vi "Cycling_No_DAQ_Tasks_RT - .5C - Test.vi"() -> ()   [LabVIEW 2020]
panel:
  out "PS Visa Out 3":refnum<visa-resource-name>
  out "PS error out 3":errorcluster
  in  "PS error in 3":errorcluster caption="PS error in (no error)"
  out "PS Visa Out 2":refnum<visa-resource-name>
  out "PS error out 2":errorcluster
  in  "PS error in 2":errorcluster caption="PS error in (no error)"
  out "PS error out":errorcluster
  out "PS Visa Out":refnum<visa-resource-name>
  in  "PS error in":errorcluster caption="PS error in (no error)"
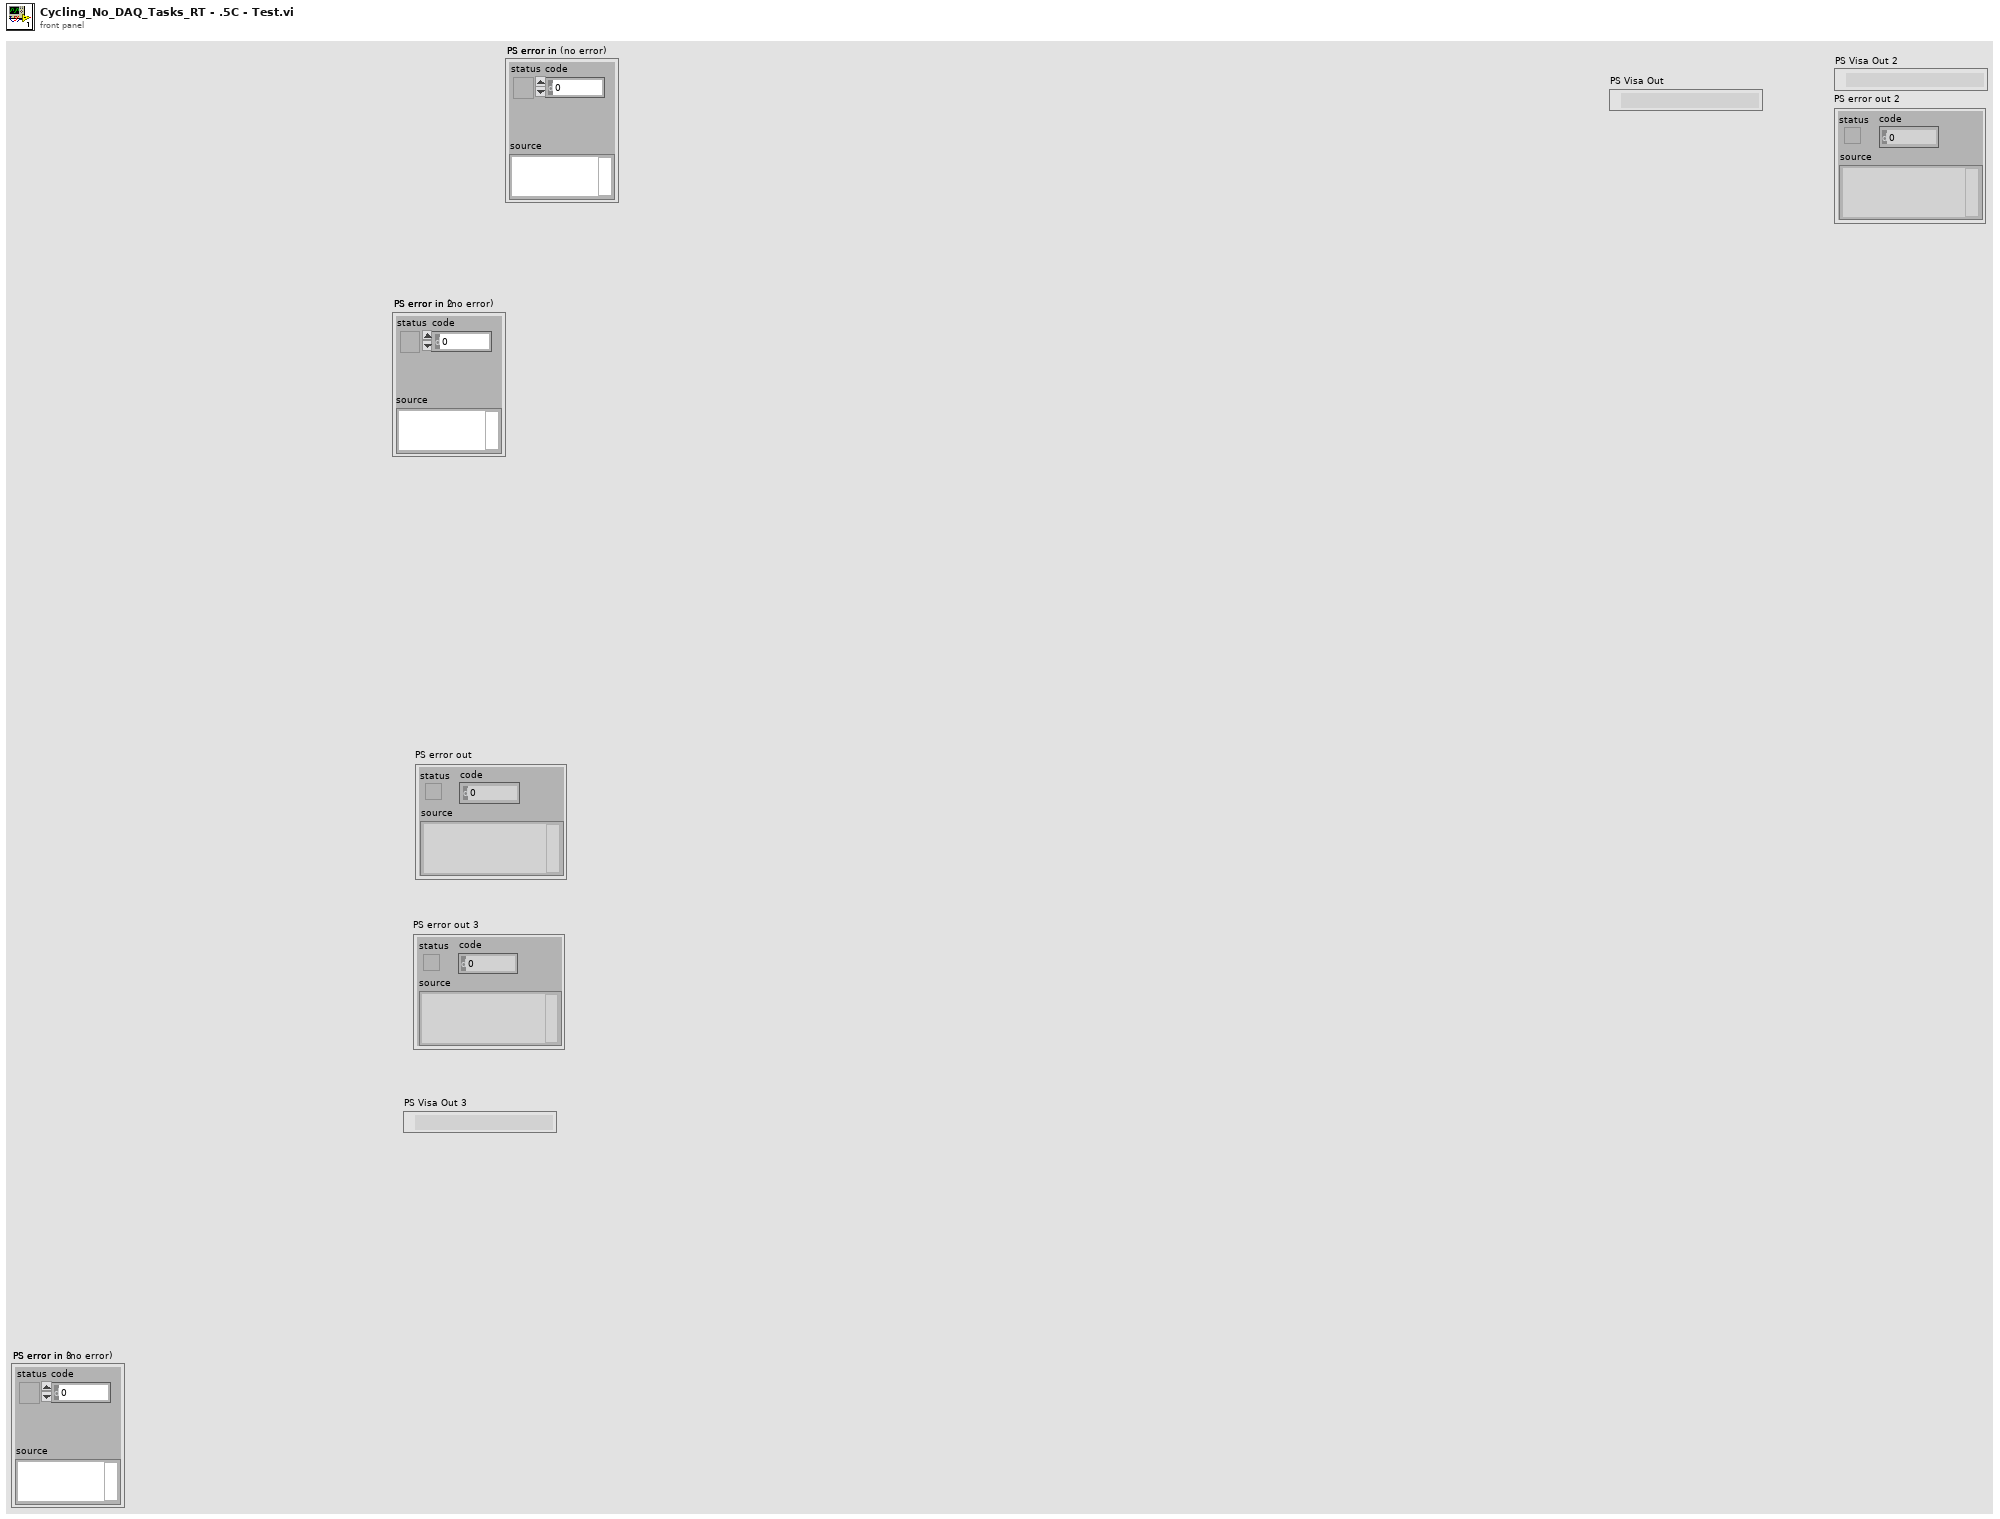
[diagram p1: front panel]
types:
  T1 = enum16{"\"30Q\"", "\"40T\"", "\"2P30Q\"", "\"3P30Q\"", "\"Nissan Leaf\""}
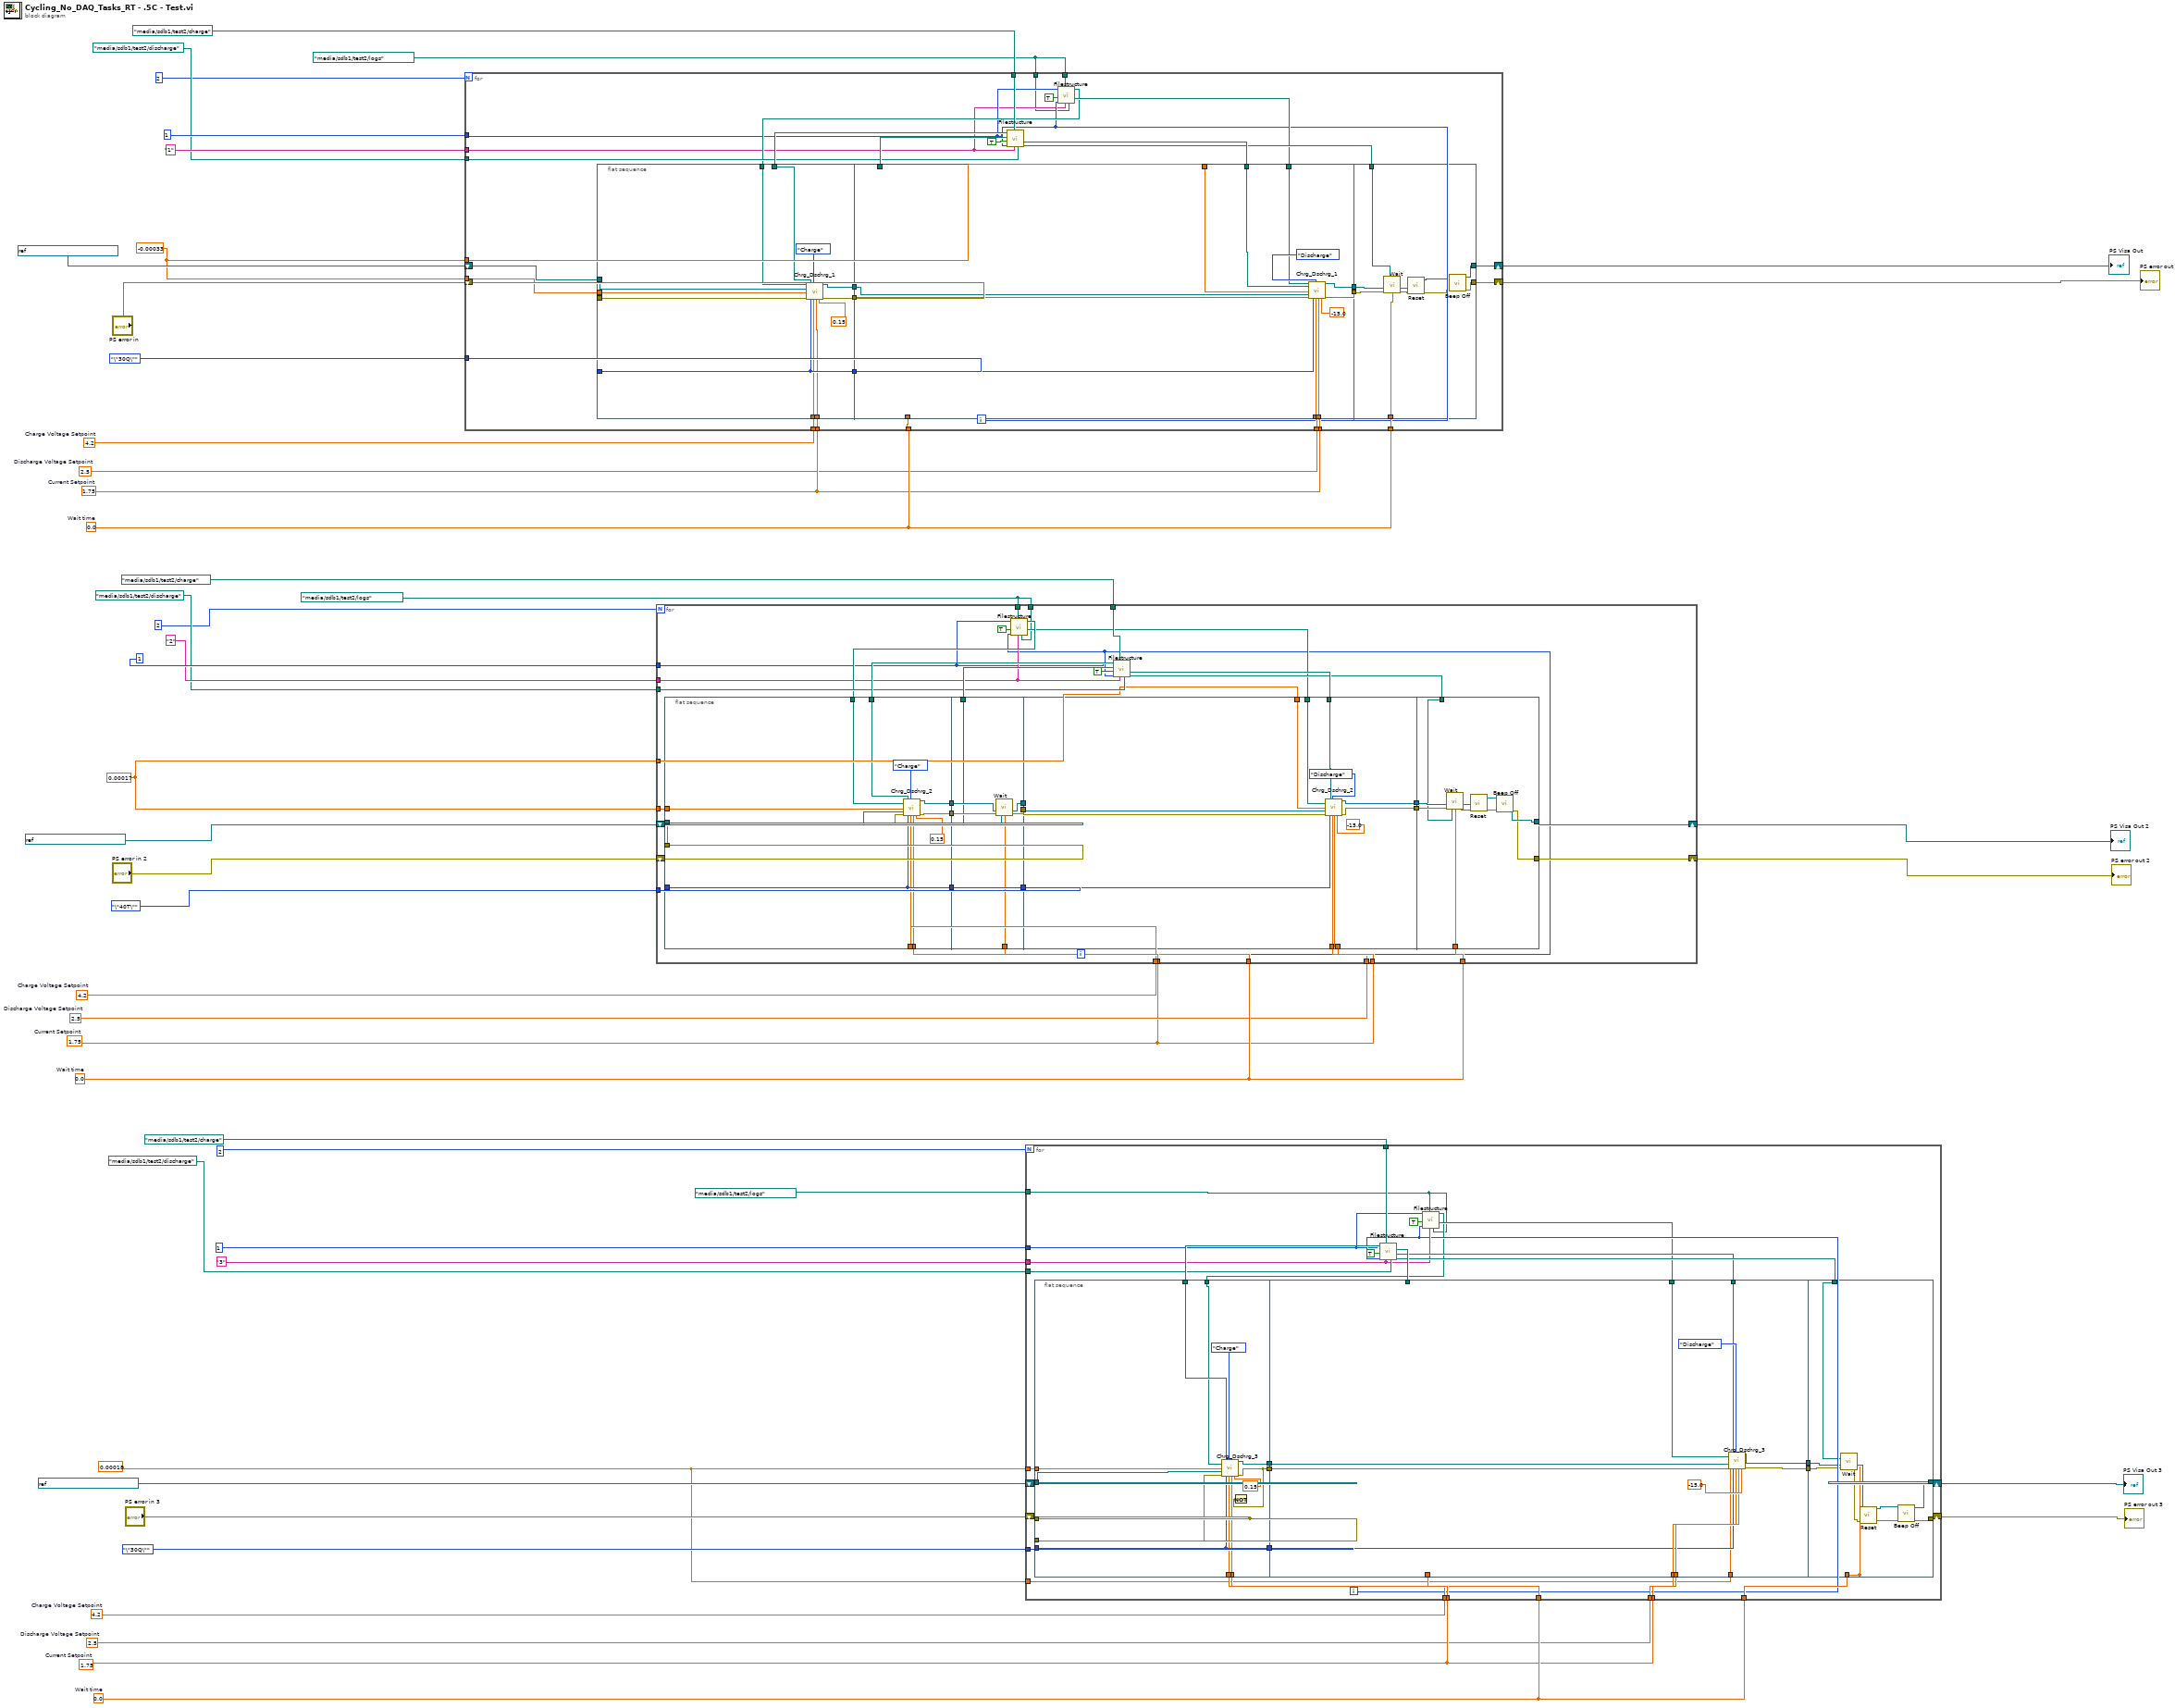
[diagram p0: block diagram]
diagram:
  w2 = path "/media/sdb1/test2/logs" ("Error log filepath")
  w3 = path "/media/sdb1/test2/logs" ("Error log filepath")
  w4 = 0.00018 ("Strain Offset")
  w5 = 0.00017 ("Strain Offset")
  w6 = 2.5  # Discharge Voltage Setpoint
  w9 = 0.0  # Wait time
  w7 = 1.75  # Current Setpoint
  w8 = 4.2  # Charge Voltage Setpoint
  w12 = 2.5  # Discharge Voltage Setpoint
  w13 = 0.0  # Wait time
  w11 = 1.75  # Current Setpoint
  w10 = 4.2  # Charge Voltage Setpoint
  w14 = 2.5  # Discharge Voltage Setpoint
  w17 = -0.00033 ("Strain Offset")
  w18 = 0.0  # Wait time
  w16 = 1.75  # Current Setpoint
  w15 = 4.2  # Charge Voltage Setpoint
  n1 = for {
    N: 2 ("Number of Cycles") -> [_]
    tunnel: T1."\"30Q\"" ("Battery Type") -> [w74]
    tunnel: w15 -> [w73]
    tunnel: w16 -> [w72]
    tunnel: w18 -> [w63]
    shift-right: [w58] -> w45
    shift-left: refnum<visa-resource-name> "TCPIP0::192.168.0.246::inst0::INSTR" ("PS VISA in") -> [w76]
    shift-right: [w57] -> w46
    shift-left: "PS error in" -> [w75]
    tunnel: 1 ("Starting Cycle") -> [w51]
    tunnel: "1" ("Batteryname") -> [w50]
    tunnel: path "/media/sdb1/test2/discharge" ("Discharge filepath") -> [w66]
    tunnel: path "/media/sdb1/test2/charge" ("Charge filepath") -> [w65]
    tunnel: w18 -> [w64]
    tunnel: w17 -> [w62]
    tunnel: w17 -> [w61]
    tunnel: w16 -> [w60]
    tunnel: w14 -> [w59]
    tunnel: w2 -> [w55]
    tunnel: w2 -> [w49]
    i -> [w52]
    n2 = flat-sequence {
      tunnel: w76 -> [w87]
      tunnel: w75 -> [w88]
      tunnel: w74 -> [w89]
      tunnel: w73 -> [w84]
      tunnel: [w91] -> w81
      tunnel: [w83] -> w80
      tunnel: [w89] -> w79
      tunnel: w71 -> [w92]
      tunnel: w62 -> [w86]
      tunnel: w60 -> [w85]
      tunnel: w53 -> [w82]
      tunnel: w59 -> [w103]
      tunnel: w72 -> [w104]
      tunnel: w69 -> [w101]
      tunnel: [w99] -> w78
      tunnel: [w98] -> w77
      tunnel: w61 -> [w97]
      tunnel: w54 -> [w96]
      tunnel: w63 -> [_]
      tunnel: w70 -> [_]
      tunnel: w79 -> [w102]
      tunnel: w80 -> [w94]
      tunnel: w81 -> [w95]
      tunnel: w68 -> [w110]
      tunnel: w78 -> [w115]
      tunnel: w77 -> [w114]
      tunnel: w64 -> [w111]
      tunnel: [w107] -> w58
      tunnel: [w106] -> w57
      frame #0 {
        n3 = call "Chrg_Dschrg_1.vi"("Error log filepath"=w82, "Strain Offset"=w86, "PS VISA in"=w87, "PS error in"=w88, "CyclePath"=w92, "Battery Type"=w89, "Charge/discharge"=enum8{"Charge", "Discharge"}."Charge", "Charge/Discharge Voltage Setpoint"=w84, "Current Setpoint"=w85, "Current Cutoff"=0.15) -> ("PS VISA out"=w91:refnum<visa-resource-name>, "PS error out"=w83:errorcluster)  [unwired: 8 in]
      }
      frame #1 {
        n4 = call "Chrg_Dschrg_1.vi"("Error log filepath"=w96, "Strain Offset"=w97, "PS VISA in"=w95, "PS error in"=w94, "CyclePath"=w101, "Battery Type"=w102, "Charge/discharge"=enum8{"Charge", "Discharge"}."Discharge", "Charge/Discharge Voltage Setpoint"=w103, "Current Setpoint"=w104, "Current Cutoff"=-15.0) -> ("PS VISA out"=w99:refnum<visa-resource-name>, "PS error out"=w98:errorcluster)  [unwired: 8 in]
      }
      frame #2 {
        n5 = call "Wait.vi"("PS VISA in"=w115, "PS error in"=w114, "Wait Filepath"=w110, "Wait time"=w111) -> ("PS Visa Out"=w113:refnum<visa-resource-name>, "PS error out"=w112:errorcluster)  [unwired: 10 in]
        n6 = call "Reset.vi"("error in"=w112, "VISA resource name"=w113) -> ("error out"=w108:errorcluster, "VISA resource name out"=w109:refnum<visa-resource-name>)  [unwired: 8 in]
        n7 = call "Beep Off.vi"("error in"=w108, "VISA resource name"=w109) -> ("error out"=w106:errorcluster, "VISA resource name out"=w107:refnum<visa-resource-name>)  [unwired: 8 in]
      }
    }
    n8 = call "Filestructure.vi"("Discharge filepath"=w66, "Batteryname"=w50, "Charge filepath"=w65, "For loop i"=w52, "In for loop"=TRUE, "Starting Cycle"=w51) -> ("DischargeWaitPath"=w68:path, "DischargeCyclePath"=w69:path, "ChargeWaitPath"=w70:path, "ChargeCyclePath"=w71:path)  [unwired: 1 in, 1 out]
    n9 = call "Filestructure.vi"("Discharge filepath"=w49, "Batteryname"=w50, "Charge filepath"=w55, "For loop i"=w52, "In for loop"=TRUE, "Starting Cycle"=w51) -> ("DischargeCyclePath"=w54:path, "ChargeCyclePath"=w53:path)  [unwired: 1 in, 3 out]
  }
  "PS error out" <- w46
  "PS Visa Out" <- w45
  n10 = for {
    N: 2 ("Number of Cycles") -> [_]
    tunnel: T1."\"40T\"" ("Battery Type") -> [w141]
    tunnel: w11 -> [w140]
    tunnel: w11 -> [w139]
    shift-right: [w134] -> w35
    shift-left: refnum<visa-resource-name> "TCPIP0::192.168.0.247::inst0::INSTR" ("PS VISA in") -> [w143]
    shift-right: [w130] -> w36
    shift-left: "PS error in 2" -> [w142]
    tunnel: 1 ("Starting Cycle") -> [w119]
    tunnel: "2" ("Batteryname 2") -> [w120]
    tunnel: path "/media/sdb1/test2/discharge" ("Discharge filepath") -> [w132]
    tunnel: path "/media/sdb1/test2/charge" ("Charge filepath") -> [w131]
    tunnel: w13 -> [w129]
    tunnel: w13 -> [w128]
    tunnel: w12 -> [w127]
    tunnel: w10 -> [w126]
    tunnel: w5 -> [w125]
    tunnel: w5 -> [w124]
    tunnel: w3 -> [w117]
    tunnel: w3 -> [w116]
    i -> [w118]
    n11 = flat-sequence {
      tunnel: w143 -> [w157]
      tunnel: w142 -> [w158]
      tunnel: w141 -> [w159]
      tunnel: w140 -> [w160]
      tunnel: [w156] -> w151
      tunnel: [w153] -> w150
      tunnel: [w159] -> w149
      tunnel: w138 -> [w162]
      tunnel: w126 -> [w155]
      tunnel: w125 -> [w154]
      tunnel: w122 -> [w152]
      tunnel: w151 -> [w169]
      tunnel: w150 -> [w168]
      tunnel: [w164] -> w148
      tunnel: [w165] -> w147
      tunnel: w149 -> [w170]
      tunnel: [w170] -> w146
      tunnel: w137 -> [w167]
      tunnel: w128 -> [w166]
      tunnel: w148 -> [w177]
      tunnel: w147 -> [w178]
      tunnel: w146 -> [w179]
      tunnel: w127 -> [w180]
      tunnel: w139 -> [w181]
      tunnel: w136 -> [w176]
      tunnel: [w174] -> w145
      tunnel: [w173] -> w144
      tunnel: w124 -> [w172]
      tunnel: w121 -> [w171]
      tunnel: w135 -> [w187]
      tunnel: w145 -> [w192]
      tunnel: w144 -> [w191]
      tunnel: w129 -> [w188]
      tunnel: [w186] -> w134
      tunnel: [w183] -> w130
      frame #0 {
        n12 = call "Chrg_Dschrg_2.vi"("Error log filepath"=w152, "Strain Offset"=w154, "PS VISA in"=w157, "PS error in"=w158, "CyclePath"=w162, "Battery Type"=w159, "Charge/discharge"=enum8{"Charge", "Discharge"}."Charge", "Charge/Discharge Voltage Setpoint"=w155, "Current Setpoint"=w160, "Current Cutoff"=0.15) -> ("PS VISA out"=w156:refnum<visa-resource-name>, "PS error out"=w153:errorcluster)  [unwired: 8 in]
      }
      frame #1 {
        n13 = call "Wait.vi"("PS VISA in"=w169, "PS error in"=w168, "Wait Filepath"=w167, "Wait time"=w166) -> ("PS Visa Out"=w164:refnum<visa-resource-name>, "PS error out"=w165:errorcluster)  [unwired: 10 in]
      }
      frame #2 {
        n14 = call "Chrg_Dschrg_2.vi"("Error log filepath"=w171, "Strain Offset"=w172, "PS VISA in"=w177, "PS error in"=w178, "CyclePath"=w176, "Battery Type"=w179, "Charge/discharge"=enum8{"Charge", "Discharge"}."Discharge", "Charge/Discharge Voltage Setpoint"=w180, "Current Setpoint"=w181, "Current Cutoff"=-15.0) -> ("PS VISA out"=w174:refnum<visa-resource-name>, "PS error out"=w173:errorcluster)  [unwired: 8 in]
      }
      frame #3 {
        n15 = call "Wait.vi"("PS VISA in"=w192, "PS error in"=w191, "Wait Filepath"=w187, "Wait time"=w188) -> ("PS Visa Out"=w190:refnum<visa-resource-name>, "PS error out"=w189:errorcluster)  [unwired: 10 in]
        n16 = call "Reset.vi"("error in"=w189, "VISA resource name"=w190) -> ("error out"=w184:errorcluster, "VISA resource name out"=w185:refnum<visa-resource-name>)  [unwired: 8 in]
        n17 = call "Beep Off.vi"("error in"=w184, "VISA resource name"=w185) -> ("error out"=w183:errorcluster, "VISA resource name out"=w186:refnum<visa-resource-name>)  [unwired: 8 in]
      }
    }
    n18 = call "Filestructure.vi"("Discharge filepath"=w116, "Batteryname"=w120, "Charge filepath"=w117, "For loop i"=w118, "In for loop"=TRUE, "Starting Cycle"=w119) -> ("DischargeCyclePath"=w121:path, "ChargeCyclePath"=w122:path)  [unwired: 1 in, 3 out]
    n19 = call "Filestructure.vi"("Discharge filepath"=w132, "Batteryname"=w120, "Charge filepath"=w131, "For loop i"=w118, "In for loop"=TRUE, "Starting Cycle"=w119) -> ("DischargeWaitPath"=w135:path, "DischargeCyclePath"=w136:path, "ChargeWaitPath"=w137:path, "ChargeCyclePath"=w138:path)  [unwired: 1 in, 1 out]
  }
  "PS error out 2" <- w36
  "PS Visa Out 2" <- w35
  n20 = for {
    N: 2 ("Number of Cycles") -> [_]
    tunnel: T1."\"30Q\"" ("Battery Type") -> [w218]
    tunnel: w7 -> [w217]
    tunnel: w7 -> [w216]
    tunnel: w9 -> [w212]
    shift-right: [w211] -> w25
    shift-left: refnum<visa-resource-name> "TCPIP0::192.168.0.248::inst0::INSTR" ("PS VISA in") -> [w219]
    shift-right: [w207] -> w26
    shift-left: "PS error in 3" -> [w202]
    tunnel: 1 ("Starting Cycle") -> [w196]
    tunnel: "3" ("Batteryname 3") -> [w198]
    tunnel: path "/media/sdb1/test2/discharge" ("Discharge filepath") -> [w209]
    tunnel: path "/media/sdb1/test2/charge" ("Charge filepath") -> [w208]
    tunnel: w9 -> [w206]
    tunnel: w8 -> [w205]
    tunnel: w6 -> [w204]
    tunnel: w4 -> [w203]
    tunnel: w4 -> [w201]
    tunnel: path "/media/sdb1/test2/logs" ("Error log filepath") -> [w193]
    i -> [w197]
    n21 = flat-sequence {
      tunnel: w219 -> [w229]
      tunnel: w202 -> [w230]
      tunnel: w218 -> [w231]
      tunnel: w217 -> [w232]
      tunnel: [w234] -> w224
      tunnel: [w226] -> w223
      tunnel: [w231] -> w222
      tunnel: w215 -> [w235]
      tunnel: w205 -> [w228]
      tunnel: w203 -> [w227]
      tunnel: w202 -> [_]
      tunnel: w194 -> [w225]
      tunnel: w204 -> [w246]
      tunnel: w216 -> [w247]
      tunnel: [w243] -> w221
      tunnel: [w242] -> w220
      tunnel: w201 -> [w241]
      tunnel: w200 -> [w240]
      tunnel: w195 -> [w239]
      tunnel: w212 -> [_]
      tunnel: w214 -> [_]
      tunnel: w222 -> [w245]
      tunnel: w223 -> [w238]
      tunnel: w224 -> [w237]
      tunnel: w213 -> [w254]
      tunnel: w221 -> [w258]
      tunnel: w220 -> [w257]
      tunnel: [w253] -> _
      tunnel: [w252] -> w211
      tunnel: [w249] -> w207
      tunnel: w206 -> [w253]
      frame #0 {
        n22 = call "Chrg_Dschrg_3.vi"("Error log filepath"=w225, "Strain Offset"=w227, "PS VISA in"=w229, "PS error in"=w230, "CyclePath"=w235, "Battery Type"=w231, "Charge/discharge"=enum8{"Charge", "Discharge"}."Charge", "Charge/Discharge Voltage Setpoint"=w228, "Current Setpoint"=w232, "Current Cutoff"=0.15) -> ("PS VISA out"=w234:refnum<visa-resource-name>, "PS error out"=w226:errorcluster)  [unwired: 8 in]
        n23 = Not(x=w226) -> ()  [unwired: 1 out]
      }
      frame #1 {
        n24 = call "Chrg_Dschrg_3.vi"("Error log filepath"=w239, "Strain Offset"=w241, "PS VISA in"=w237, "PS error in"=w238, "CyclePath"=w240, "Battery Type"=w245, "Charge/discharge"=enum8{"Charge", "Discharge"}."Discharge", "Charge/Discharge Voltage Setpoint"=w246, "Current Setpoint"=w247, "Current Cutoff"=-15.0) -> ("PS VISA out"=w243:refnum<visa-resource-name>, "PS error out"=w242:errorcluster)  [unwired: 8 in]
      }
      frame #2 {
        n25 = call "Wait.vi"("PS VISA in"=w258, "PS error in"=w257, "Wait Filepath"=w254, "Wait time"=w253) -> ("PS Visa Out"=w256:refnum<visa-resource-name>, "PS error out"=w255:errorcluster)  [unwired: 10 in]
        n26 = call "Reset.vi"("error in"=w255, "VISA resource name"=w256) -> ("error out"=w250:errorcluster, "VISA resource name out"=w251:refnum<visa-resource-name>)  [unwired: 8 in]
        n27 = call "Beep Off.vi"("error in"=w250, "VISA resource name"=w251) -> ("error out"=w249:errorcluster, "VISA resource name out"=w252:refnum<visa-resource-name>)  [unwired: 8 in]
      }
    }
    n28 = call "Filestructure.vi"("Discharge filepath"=w209, "Batteryname"=w198, "Charge filepath"=w208, "For loop i"=w197, "In for loop"=TRUE, "Starting Cycle"=w196) -> ("DischargeWaitPath"=w213:path, "DischargeCyclePath"=w200:path, "ChargeWaitPath"=w214:path, "ChargeCyclePath"=w215:path)  [unwired: 1 in, 1 out]
    n29 = call "Filestructure.vi"("Discharge filepath"=w193, "Batteryname"=w198, "Charge filepath"=w193, "For loop i"=w197, "In for loop"=TRUE, "Starting Cycle"=w196) -> ("DischargeCyclePath"=w195:path, "ChargeCyclePath"=w194:path)  [unwired: 1 in, 3 out]
  }
  "PS error out 3" <- w26
  "PS Visa Out 3" <- w25
